vi "Create.vi"(10 "Data":T1) -> (3 "History Data Value out":refnum<class "Unix ns Data Value.lvclass">)   [LabVIEW 2020, in "VolatusHistorian.lvlib" / "Unix ns Data Value.lvclass"]
uses:
  Unix ns Data Value.lvclass
  History Data (unix ns).ctl
  Channel History (unix ns).ctl
  Unix ns Data Value.lvclass/Unix ns Data Value.ctl
  VolatusHistorian.lvlib
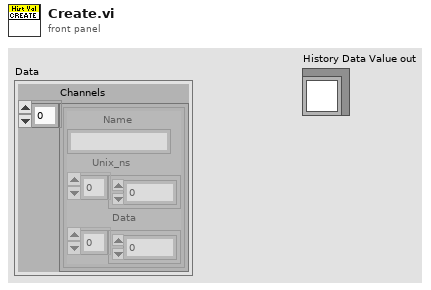
[diagram p1: front panel]
types:
  T1 = typedef "VolatusHistorian.lvlib/History Data (unix ns).ctl" = cluster{"Channels":T2[]}
  T2 = typedef "VolatusHistorian.lvlib/Channel History (unix ns).ctl" = cluster{"Name":string, "Unix_ns":i64[], "Data":dbl[]}
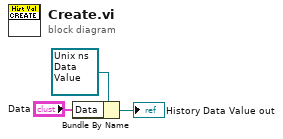
[diagram p0: block diagram]
diagram:
  n1 = Bundle By Name(cluster=refnum<class "Unix ns Data Value.lvclass"> refnum ("History Data Value in"), "Data"="Data") -> (→"History Data Value out":refnum<class "Unix ns Data Value.lvclass">)
